vi "List Open Files.vi"(8 "error in (no error)":errorcluster, 11 "Application refnum":refnum<k7>) -> (0 "error out":errorcluster, 2 "Name":string[](array[string]), 3 "Application refnum out":refnum<k7>)   [LabVIEW 2018, in "lpptx.lvlib"]
uses:
  lpptx.lvlib
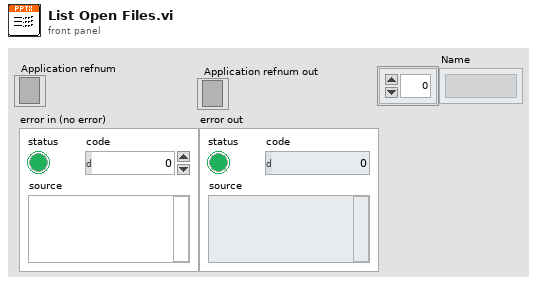
[diagram p1: front panel]
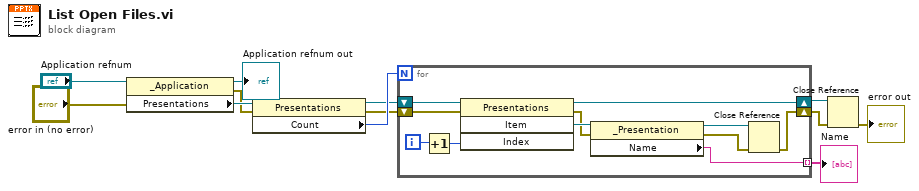
[diagram p0: block diagram]
diagram:
  n1 = property class="_Application"(reference="Application refnum", error in="error in (no error)") -> (reference out=→"Application refnum out":refnum<k7>, error out=w10:errorcluster, "Presentations"=w11:refnum<k7>)
  n2 = property class="Presentations"(reference=w11, error in=w10) -> (reference out=w8:refnum<k7>, error out=w7:errorcluster, "Count"=w9:i32)
  n3 = for {
    N: w9 -> [_]
    shift-right: [w15] -> w5
    shift-left: w7 -> [w23]
    shift-right: [w21] -> w6
    shift-left: w8 -> [w22]
    tunnel: [w16] -> w2 mode=indexing
    i -> [w14]
    n4 = Increment(x=w14) -> (x+1=w13:i32)
    n5 = invoke class="Presentations" method="Item"(reference=w22, error in=w23, "Index"=w13) -> (reference out=w21:refnum<k7>, error out=w19:errorcluster, "Item"=w20:refnum<k7>)  [unwired: 1 in, 1 out]
    n6 = property class="_Presentation"(reference=w20, error in=w19) -> (reference out=w17:refnum<k7>, error out=w18:errorcluster, "Name"=w16:string)
    n7 = Close Reference(reference=w17, error in (no error)=w18) -> (error out=w15:errorcluster)
  }
  "Name" <- w2
  n8 = Close Reference(reference=w6, error in (no error)=w5) -> (error out=→"error out":errorcluster)
